vi "main.vi"() -> ()   [LabVIEW 2018]
panel:
  in  "选项卡控件":enum32{"账户", "创建", "变更", "历史变更", "标签"}(tab)
  in  "密码":string
  in  "用户名":string(combo)
  in  "关联远程仓库":bool
  in  "远程仓库":string
  in  "创建README":bool
  in  "项目描述":string
  in  "创建仓库":bool
  in  "提交":bool
  in  "版本号（标签）":string
  in  "变更信息（必填）":string
  in  "变更项":i32(listbox)
  in  "推送变更":bool
  in  "历史变更":i32(listbox)
  in  "历史标签":i32(listbox)
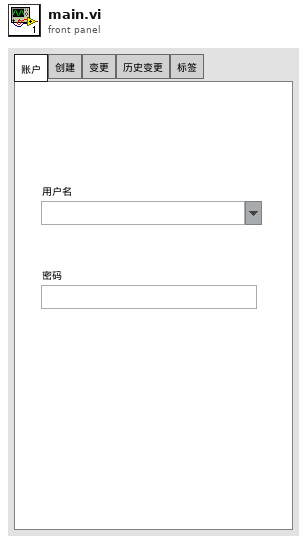
[diagram p1: front panel]
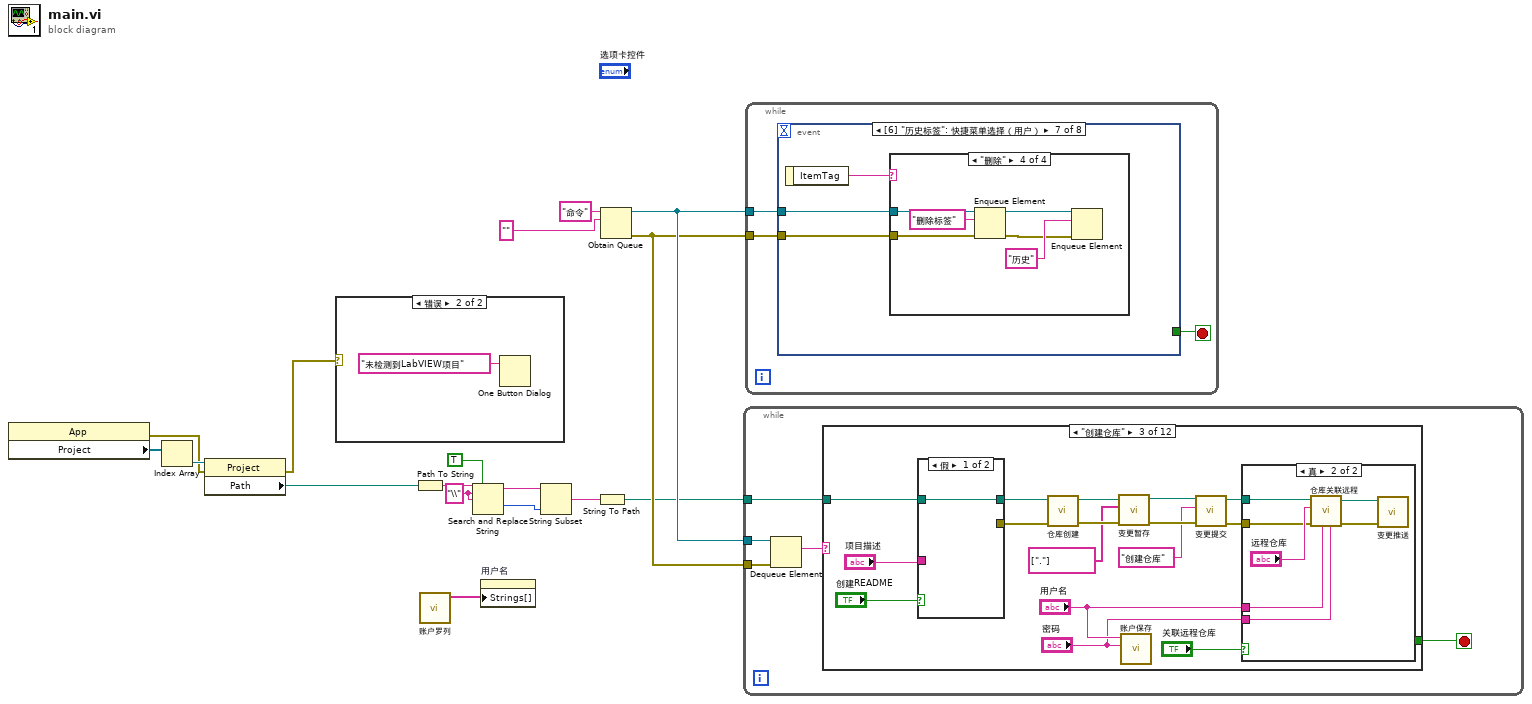
[diagram p0: block diagram]
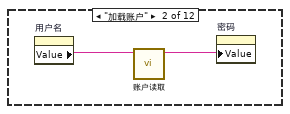
[diagram p4: hidden frame]
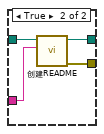
[diagram p6: hidden frame]
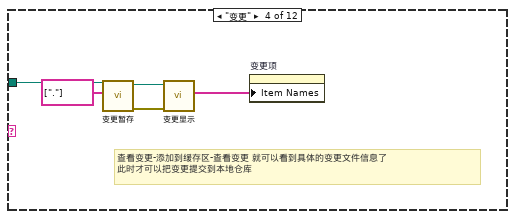
[diagram p7: hidden frame]
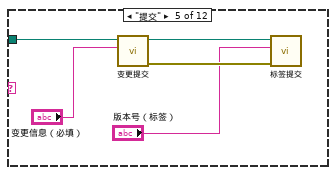
[diagram p8: hidden frame]
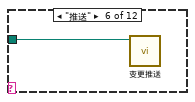
[diagram p9: hidden frame]
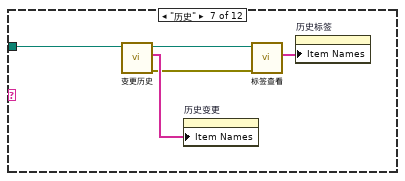
[diagram p10: hidden frame]
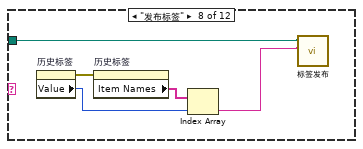
[diagram p11: hidden frame]
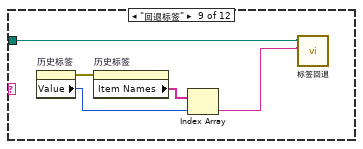
[diagram p12: hidden frame]
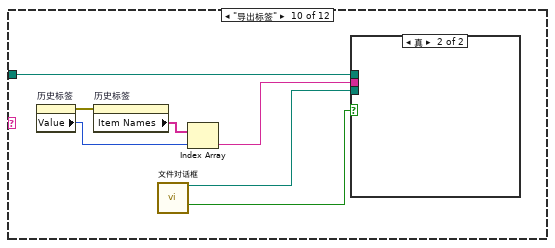
[diagram p13: hidden frame]
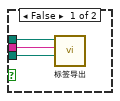
[diagram p14: hidden frame]
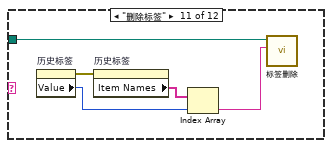
[diagram p15: hidden frame]
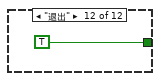
[diagram p16: hidden frame]
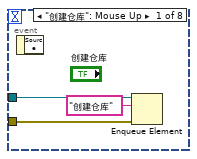
[diagram p17: hidden frame]
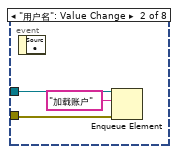
[diagram p18: hidden frame]
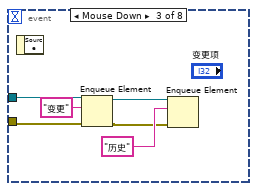
[diagram p19: hidden frame]
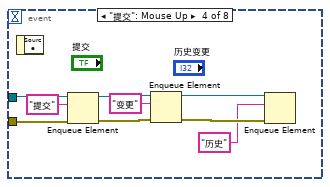
[diagram p20: hidden frame]
diagram:
  w6 = "\\" ("搜索字符串")
  n1 = property class="App"() -> (error out=w10:errorcluster, "Project"=w12:refnum<vi>[])  [unwired: 2 in, 1 out]
  n2 = Index Array(array=w12) -> (element=w11:refnum<vi>)  [unwired: 1 in]
  n3 = property class="Project"(reference=w11, error in=w10) -> (error out=w1:errorcluster, "Path"=w9:path)  [unwired: 1 out]
  n4 = case shown="错误" w1 {
    frame No Error {
    }
    frame Error {
      n5 = One Button Dialog(message="未检测到LabVIEW项目" ("消息")) -> ()  [unwired: 1 in, 1 out]
    }
  }
  n6 = Path To String(path=w9) -> (string=w8:string)
  n7 = call "账户罗列.vi"() -> ("账户名"=w13:string[])  [unwired: 10 in, 1 out]
  n8 = Search and Replace String(replace all?=TRUE ("替换全部？(F)"), input string=w8, search string=w6, replace string=w6) -> (result string=w5:string, offset past replacement=w3:i32)  [unwired: 4 in, 2 out]
  n9 = property on="用户名" class="CmbBox"("Strings[]"=w13) -> ()  [unwired: 2 in, 2 out]
  n10 = String Subset(string=w5, length (rest)=w3) -> (substring=w4:string)  [unwired: 1 in]
  n11 = String To Path(string=w4) -> (path=w2:path)
  n12 = Obtain Queue(name (unnamed)="命令" ("名称（未命名）"), element data type="") -> (queue out=w15:refnum<queue>, error out=w14:errorcluster)  [unwired: 3 in, 1 out]
  n13 = while {
    tunnel: w15 -> [w23]
    tunnel: w14 -> [w22]
    tunnel: w2 -> [w19]
    stop <- w20 stop-if-true
    n14 = Dequeue Element(queue=w23, error in (no error)=w22) -> (element=w21:string)  [unwired: 1 in, 3 out]
    n15 = case shown="\"创建仓库\"" w21 {
      tunnel: w19 -> [_ _ w36 w58 w63 w64 w69 w71 w76 w83 w94 _]
      tunnel: [_ _ _ _ _ _ _ _ _ _ _ TRUE] -> w20
      frame "null", Default {
      }
      frame "加载账户" {
        n16 = property on="用户名" class="CmbBox"() -> ("Value"=w25:string)  [unwired: 2 in, 2 out]
        n17 = call "账户读取.vi"("账户名"=w25) -> ("密码"=w24:string)  [unwired: 9 in, 1 out]
        n18 = property on="密码" class="Str"("Value"=w24) -> ()  [unwired: 2 in, 2 out]
      }
      frame "创建仓库" {
        n19 = case shown="假" "创建README" {
          tunnel: "项目描述" -> [_ w53]
          tunnel: [_ w52] -> w34
          tunnel: w36 -> [w49 w51]
          tunnel: [w49 w50] -> w35
          frame False {
          }
          frame True {
            n20 = call "创建README.vi"("描述"=w53, "基路径"=w51) -> ("错误输出"=w52:errorcluster, "基路径"=w50:path)  [unwired: 8 in]
          }
        }
        n21 = call "仓库创建.vi"("error in"=w34, "仓库路径"=w35) -> ("error out"=w32:errorcluster, "仓库路径"=w33:path)  [unwired: 6 in, 2 out]
        n22 = call "变更暂存.vi"("error in"=w32, "变更项"=string[] ["."], "仓库路径"=w33) -> ("error out"=w38:errorcluster, "仓库路径"=w39:path)  [unwired: 5 in, 2 out]
        n23 = call "账户保存.vi"("密码"="密码", "账户名"="用户名") -> ()  [unwired: 9 in, 1 out]
        n24 = call "变更提交.vi"("error in"=w38, "变更信息"="创建仓库", "仓库路径"=w39) -> ("error out"=w29:errorcluster, "仓库路径"=w30:path)  [unwired: 5 in, 2 out]
        n25 = case shown="真" "关联远程仓库" {
          tunnel: w30 -> [_ w48]
          tunnel: w29 -> [_ w46]
          tunnel: "用户名" -> [_ w43]
          tunnel: "密码" -> [_ w42]
          frame False {
          }
          frame True {
            n26 = call "仓库关联远程.vi"("密码"=w42, "用户名"=w43, "error in"=w46, "远程仓库"="远程仓库", "仓库路径"=w48) -> ("error out"=w44:errorcluster, "仓库路径"=w45:path)  [unwired: 3 in, 2 out]
            n27 = call "变更推送.vi"("error in"=w44, "仓库路径"=w45) -> ()  [unwired: 6 in, 4 out]
          }
        }
      }
      frame "变更" {
        # "查看变更-添加到缓存区-查看变更 就可以看到具体的变更文件信息了\n此时才可以把变更提交到本地仓库"
        n28 = call "变更暂存.vi"("变更项"=string[] ["."], "仓库路径"=w58) -> ("error out"=w57:errorcluster, "仓库路径"=w56:path)  [unwired: 6 in, 2 out]
        n29 = call "变更显示.vi"("error in"=w57, "仓库路径"=w56) -> ("变更项"=w55:string[])  [unwired: 6 in, 3 out]
        n30 = property on="变更项" class="LstBox (严格)"("Item Names"=w55) -> ()  [unwired: 2 in, 2 out]
      }
      frame "提交" {
        n31 = call "变更提交.vi"("变更信息"="变更信息（必填）", "仓库路径"=w63) -> ("error out"=w60:errorcluster, "仓库路径"=w61:path)  [unwired: 6 in, 2 out]
        n32 = call "标签提交.vi"("error in"=w60, "标签（版本）"="版本号（标签）", "仓库路径"=w61) -> ()  [unwired: 5 in, 4 out]
      }
      frame "推送" {
        n33 = call "变更推送.vi"("仓库路径"=w64) -> ()  [unwired: 7 in, 4 out]
      }
      frame "历史" {
        n34 = call "变更历史.vi"("仓库路径"=w69) -> ("error out"=w66:errorcluster, "变更项"=w68:string[], "仓库路径"=w67:path)  [unwired: 7 in, 1 out]
        n35 = property on="历史变更" class="LstBox (严格)"("Item Names"=w68) -> ()  [unwired: 2 in, 2 out]
        n36 = call "标签查看.vi"("error in"=w66, "仓库路径"=w67) -> ("standard output"=w65:string[])  [unwired: 6 in, 3 out]
        n37 = property on="历史标签" class="LstBox (严格)"("Item Names"=w65) -> ()  [unwired: 2 in, 2 out]
      }
      frame "发布标签" {
        n38 = property on="历史标签" class="LstBox (严格)"() -> (error out=w74:errorcluster, "Value"=w72:i32)  [unwired: 2 in, 1 out]
        n39 = property on="历史标签" class="LstBox (严格)"(error in=w74) -> ("Item Names"=w73:string[])  [unwired: 1 in, 2 out]
        n40 = Index Array(array=w73, index=w72) -> (element=w70:string)
        n41 = call "标签发布.vi"("标签（版本）"=w70, "仓库路径"=w71) -> ()  [unwired: 6 in, 4 out]
      }
      frame "回退标签" {
        n42 = property on="历史标签" class="LstBox (严格)"() -> (error out=w79:errorcluster, "Value"=w77:i32)  [unwired: 2 in, 1 out]
        n43 = property on="历史标签" class="LstBox (严格)"(error in=w79) -> ("Item Names"=w78:string[])  [unwired: 1 in, 2 out]
        n44 = Index Array(array=w78, index=w77) -> (element=w75:string)
        n45 = call "标签回退.vi"("标签（版本）"=w75, "仓库路径"=w76) -> ()  [unwired: 6 in, 4 out]
      }
      frame "导出标签" {
        n46 = property on="历史标签" class="LstBox (严格)"() -> (error out=w86:errorcluster, "Value"=w84:i32)  [unwired: 2 in, 1 out]
        n47 = property on="历史标签" class="LstBox (严格)"(error in=w86) -> ("Item Names"=w85:string[])  [unwired: 1 in, 2 out]
        n48 = call "文件对话框"() -> ("selected path"=w81:path, "cancelled"=w80:bool)  [unwired: 12 in, 2 out]
        n49 = Index Array(array=w85, index=w84) -> (element=w82:string)
        n50 = case shown="真" w80 {
          tunnel: w83 -> [w89 _]
          tunnel: w82 -> [w88 _]
          tunnel: w81 -> [w87 _]
          frame False {
            n51 = call "标签导出.vi"("目标仓库"=w87, "标签（版本）"=w88, "仓库路径"=w89) -> ()  [unwired: 5 in, 4 out]
          }
          frame True {
          }
        }
      }
      frame "删除标签" {
        n52 = property on="历史标签" class="LstBox (严格)"() -> (error out=w93:errorcluster, "Value"=w91:i32)  [unwired: 2 in, 1 out]
        n53 = property on="历史标签" class="LstBox (严格)"(error in=w93) -> ("Item Names"=w92:string[])  [unwired: 1 in, 2 out]
        n54 = Index Array(array=w92, index=w91) -> (element=w90:string)
        n55 = call "标签删除.vi"("标签（版本）"=w90, "仓库路径"=w94) -> ()  [unwired: 6 in, 4 out]
      }
      frame "退出" {
      }
    }
  }
  n56 = while {
    tunnel: w15 -> [w98]
    tunnel: w14 -> [w97]
    stop <- w96 stop-if-true
    n57 = event shown="[6] \"历史标签\": 快捷菜单选择（用户）" {
      selector: _ -> [_ _ _ _ _ _ _ _]
      dyn-events: _ -> [_ _ _ _ _ _ _ _]
      timeout: _ -> [_ _ _ _ _ _ _ _]
      tunnel: w98 -> [w101 w104 w110 w119 w122 _ w128 w148]
      tunnel: w97 -> [w100 w103 w109 w118 w121 _ w127 w147]
      tunnel: [_ _ _ _ _ _ _ TRUE] -> w96
      event "创建仓库": Mouse Up {
        n58 = event-data() -> ()  [unwired: 1 in, 1 out]
        n59 = Enqueue Element(queue=w101, element="创建仓库" ("元素"), error in (no error)=w100) -> ()  [unwired: 1 in, 3 out]
      }
      event "用户名": Value Change {
        n60 = event-data() -> ()  [unwired: 1 in, 1 out]
        n61 = Enqueue Element(queue=w104, element="加载账户" ("元素"), error in (no error)=w103) -> ()  [unwired: 1 in, 3 out]
      }
      event Mouse Down {
        n62 = event-data() -> ()  [unwired: 1 in, 1 out]
        n63 = Enqueue Element(queue=w110, element="变更" ("元素"), error in (no error)=w109) -> (queue out=w105:refnum<queue>, error out=w106:errorcluster)  [unwired: 1 in, 1 out]
        n64 = Enqueue Element(queue=w105, element="历史" ("元素"), error in (no error)=w106) -> ()  [unwired: 1 in, 3 out]
      }
      event "提交": Mouse Up {
        n65 = event-data() -> ()  [unwired: 1 in, 1 out]
        n66 = Enqueue Element(queue=w119, element="提交" ("元素"), error in (no error)=w118) -> (queue out=w112:refnum<queue>, error out=w111:errorcluster)  [unwired: 1 in, 1 out]
        n67 = Enqueue Element(queue=w112, element="变更" ("元素"), error in (no error)=w111) -> (queue out=w115:refnum<queue>, error out=w116:errorcluster)  [unwired: 1 in, 1 out]
        n68 = Enqueue Element(queue=w115, element="历史" ("元素"), error in (no error)=w116) -> ()  [unwired: 1 in, 3 out]
      }
      event "推送变更": Mouse Up {
        n69 = event-data() -> ()  [unwired: 1 in, 1 out]
        n70 = Enqueue Element(queue=w122, element="推送" ("元素"), error in (no error)=w121) -> ()  [unwired: 1 in, 3 out]
      }
      event "历史标签": Shortcut Menu Activation? {
        n71 = event-data() -> ("MenuRef"=w126:refnum<k9>)  [unwired: 1 in]
        n72 = Delete Menu Items(9:w126) -> (0:w123:errorcluster, 3:w125:refnum<k9>)  [unwired: 3 in]
        n73 = Insert Menu Items(6:w123, 7:string[] ["发布", "回退", "导出", "删除"] ("项标识符"), 9:w125) -> ()  [unwired: 3 in, 3 out]
        n74 = event-data() -> ()  [unwired: 2 in, 1 out]
      }
      event "历史标签": Shortcut Menu Selection (User) {
        n75 = event-data() -> ("ItemTag"=w129:string)  [unwired: 1 in]
        n76 = case shown="\"删除\"" w129 {
          tunnel: w128 -> [w131 w134 w138 w144]
          tunnel: w127 -> [w130 w133 w137 w143]
          frame "发布", Default {
            n77 = Enqueue Element(queue=w131, element="发布标签" ("元素"), error in (no error)=w130) -> ()  [unwired: 1 in, 3 out]
          }
          frame "回退" {
            n78 = Enqueue Element(queue=w134, element="回退标签" ("元素"), error in (no error)=w133) -> ()  [unwired: 1 in, 3 out]
          }
          frame "导出" {
            n79 = Enqueue Element(queue=w138, element="导出标签" ("元素"), error in (no error)=w137) -> ()  [unwired: 1 in, 3 out]
          }
          frame "删除" {
            n80 = Enqueue Element(queue=w144, element="删除标签" ("元素"), error in (no error)=w143) -> (queue out=w140:refnum<queue>, error out=w139:errorcluster)  [unwired: 1 in, 1 out]
            n81 = Enqueue Element(queue=w140, element="历史" ("元素"), error in (no error)=w139) -> ()  [unwired: 1 in, 3 out]
          }
        }
      }
      event Panel Close {
        n82 = event-data() -> ()  [unwired: 1 in, 1 out]
        n83 = Enqueue Element(queue=w148, element="退出" ("元素"), error in (no error)=w147) -> ()  [unwired: 1 in, 3 out]
      }
    }
  }
